vi "Get Attribute VAR.vi"(8 "error in":errorcluster, 9 "Data Type and Default Value":variant, 10 "Attribute":string, 11 "Config from Excel Table in":refnum<class "Config from Excel Table.lvclass">) -> (0 "error out":errorcluster, 2 "Value":variant, 3 "Config from Excel Table out":refnum<class "Config from Excel Table.lvclass">)   [LabVIEW 2019, in "Config from Excel Table.lvclass"]
uses:
  Config from Excel Table.lvclass
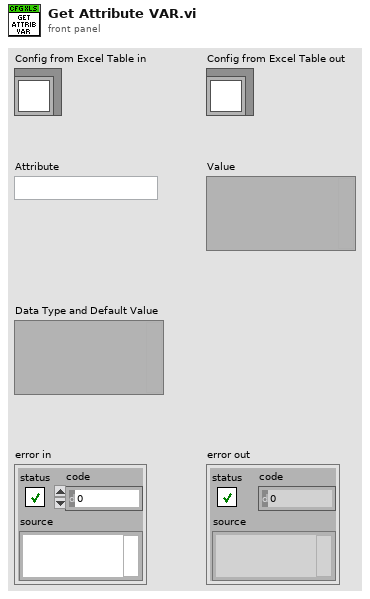
[diagram p1: front panel]
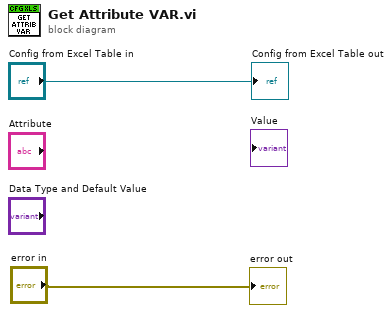
[diagram p0: block diagram]
diagram:
  "error out" <- "error in"
  "Config from Excel Table out" <- "Config from Excel Table in"
